vi "image queue to disk and to display queue_MD.vi"() -> ()   [LabVIEW 2012]
uses:
  <vilib>/Utility/VariantDataType/Type.ctl
  Custom Controls/file format type def.ctl
  GFG/GFGnumericGet.vi
  GFG/GFGbooleanGet.vi
  save images/save channels to raw bin files.vi
  save images/save channels to interleaved multi-tiff files.vi
  save images/save channels to separate multi-tiff files.vi
  save images/save channels to stacked multi-tiff files.vi
  save images/save channels to interleaved tiff series.vi
  save images/save channels to separate tiff series.vi
  save images/save channels to stacked tiff series.vi
  GFG/GFG library.lvlib
  <vilib>/Utility/VariantDataType/VariantType.lvlib
panel:
  out "error out 4":errorcluster
  out "error out 3":errorcluster
  out "error out 2":errorcluster
  out "# elements in image data queue":i32
  out "error out":errorcluster
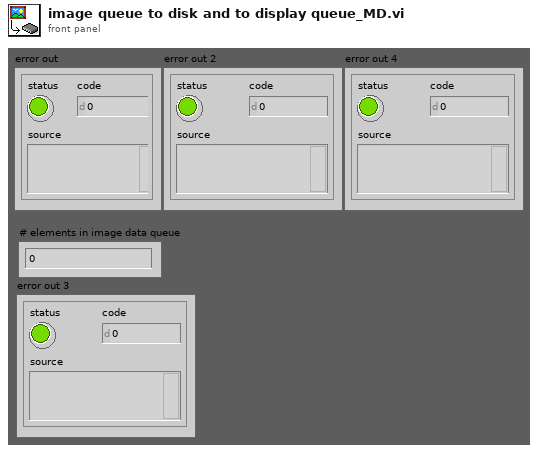
[diagram p1: front panel]
types:
  T1 = typedef "file format type def.ctl" = enum16{"16bit raw", "32bit raw", "16bit multi-tiff (interleave)", "16bit multi-tiff (separate)", "16bit multi-tiff (stacked)", "32bit multi-tiff (interleave)", "32bit multi-tiff (separate)", "32bit multi-tiff (stacked)", "16bit tiff series (interleave)", "16bit tiff series (separate)", "16bit tiff series (stacked)", "32bit tiff series (interleave)", "32bit tiff series (separate)", "32bit tiff series (stacked)"}
  T2 = cluster{"NewVal":bool, "Event Registration Refnum":refnum<event-registration>}
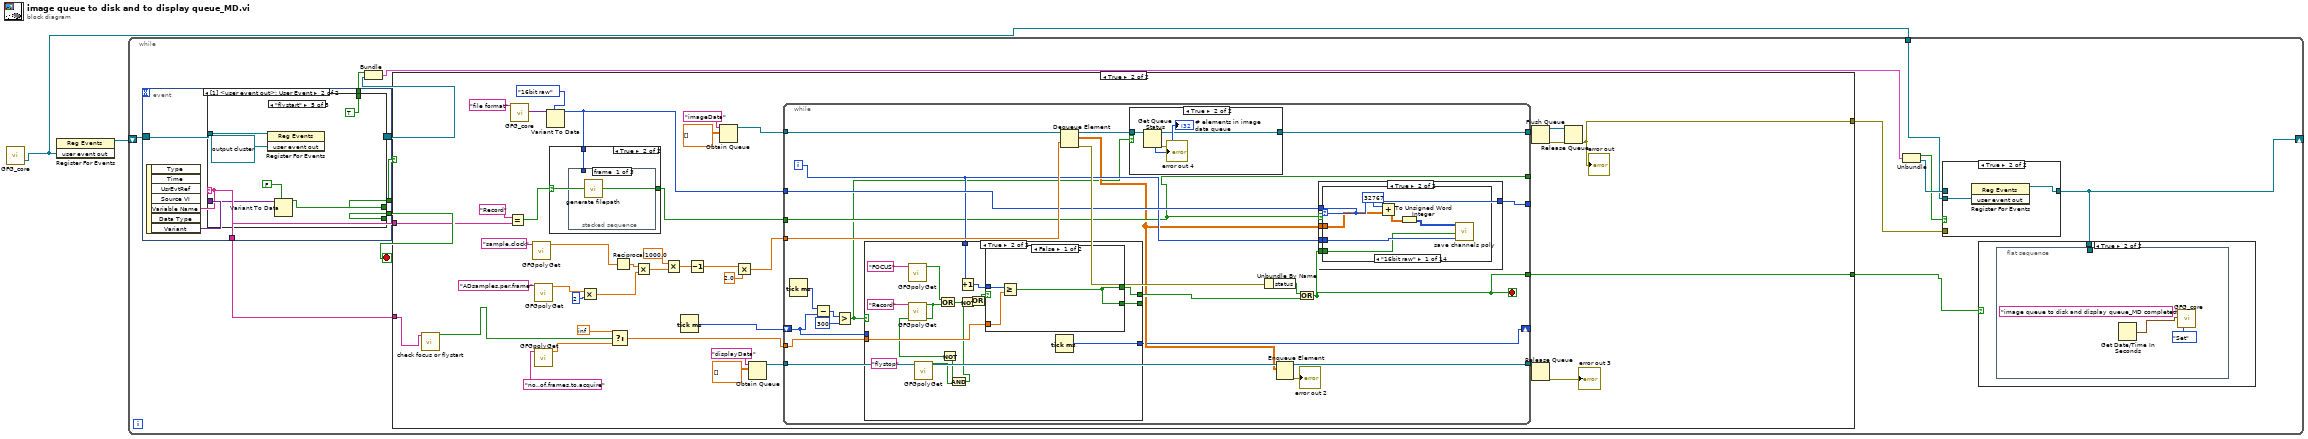
[diagram p0: block diagram]
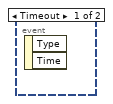
[diagram p4: hidden frame]
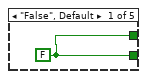
[diagram p5: hidden frame]
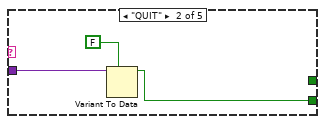
[diagram p6: hidden frame]
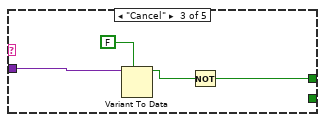
[diagram p7: hidden frame]
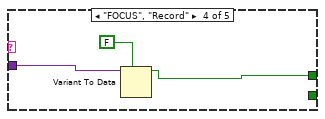
[diagram p8: hidden frame]
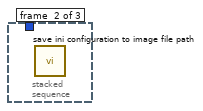
[diagram p11: hidden frame]
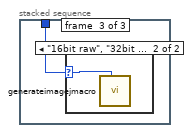
[diagram p12: hidden frame]
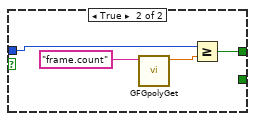
[diagram p16: hidden frame]
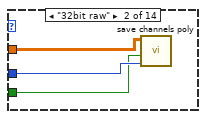
[diagram p18: hidden frame]
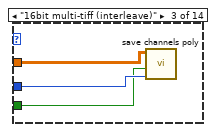
[diagram p19: hidden frame]
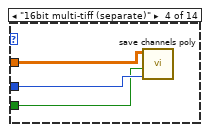
[diagram p20: hidden frame]
diagram:
  n1 = call "GFG_core.vi"() -> ("user event out"=w1:refnum<user-event>)  [unwired: 13 in, 6 out]
  n2 = register-events(w1) -> (reference out=w2:refnum<event-registration>)  [unwired: 2 in, 1 out]
  n3 = while {
    tunnel: w1 -> [w6]
    shift-right: [w4] -> _
    shift-left: w2 -> [w13]
    stop <- w15 stop-if-true
    n4 = event shown="[1] <user event out>: User Event" {
      selector: w13 -> [_ w24]
      dyn-events: [_ _] -> w11
      timeout: _ -> [_ _]
      tunnel: [_ w28] -> w14
      tunnel: [_ w27] -> w15
      tunnel: [_ w25] -> w5
      tunnel: [_ w23] -> w12
      event Timeout {
        n5 = event-data() -> ()  [unwired: 1 in, 2 out]
      }
      event User Event {
        n6 = event-data() -> ("Variable Name"=w25:string, "Variant"=w26:variant)  [unwired: 1 in, 5 out]
        n7 = case shown="\"flystart\"" w25 {
          tunnel: [w29 _ w33 w37 w43] -> w28
          tunnel: [w29 w30 _ _ _] -> w27
          tunnel: w26 -> [_ w32 w35 w38 w44]
          tunnel: w24 -> [_ _ _ _ w41]
          tunnel: [_ _ _ _ TRUE ("NewVal")] -> w23
          frame "False", Default {
            w29 = FALSE ("NewVal")
          }
          frame "QUIT" {
            n8 = Variant To Data(type=FALSE ("NewVal"), Variant=w32) -> (data=w30:bool)  [unwired: 1 in, 1 out]
          }
          frame "Cancel" {
            n9 = Variant To Data(type=FALSE ("NewVal"), Variant=w35) -> (data=w34:bool)  [unwired: 1 in, 1 out]
            n10 = Not(x=w34) -> (.not. x?=w33:bool)
          }
          frame "FOCUS", "Record" {
            n11 = Variant To Data(type=FALSE ("NewVal"), Variant=w38) -> (data=w37:bool)  [unwired: 1 in, 1 out]
          }
          frame "flystart" {
            n12 = register-events(reference=w41, refnum<user-event> refnum ("user event out")) -> ()  [unwired: 1 in, 2 out]
            n13 = Variant To Data(type=FALSE ("NewVal"), Variant=w44) -> (data=w43:bool)  [unwired: 1 in, 1 out]
          }
        }
      }
    }
    n14 = Bundle("NewVal"=w12, "Event Registration Refnum"=w11) -> (w9:T2)  [unwired: 1 in]
    n15 = case shown="True" w14 {
      tunnel: w5 -> [_ w64]
      tunnel: [_ w53] -> w10
      tunnel: w5 -> [_ w48]
      tunnel: [_ w46] -> w3
      frame False {
      }
      frame True {
        n16 = call "check focus or flystart.vi"("x"=w48) -> ("x .or. y?"=w47:bool)  [unwired: 10 in]
        n17 = Equal?(x="Record", y=w64) -> (x = y?=w58:bool)
        n18 = call "GFG_core.vi"("Variable Name in"="file format") -> ("Variant Out"=w60:variant)  [unwired: 12 in, 6 out]
        n19 = call-poly "GFGpolyGet.vi"("Variable Name in"="sample.clock" ("Tag in")) -> ("Numeric"=w71:dbl)  [unwired: 9 in, 1 out]
        n20 = call-poly "GFGpolyGet.vi"("Variable Name in"="ADsamples.per.frame" ("Tag in")) -> ("Numeric"=w77:dbl)  [unwired: 9 in, 1 out]
        n21 = call-poly "GFGpolyGet.vi"("Variable Name in"="no..of.frames.to.acquire" ("Tag in")) -> ("Numeric"=w50:dbl)  [unwired: 9 in, 1 out]
        n22 = Variant To Data(type=file_format_type_def."16bit raw" ("file format"), Variant=w60) -> (data=w56:T1)  [unwired: 1 in, 1 out]
        n23 = case shown="True" w58 {
          selector: w58 -> [w87 w89]
          tunnel: [w87 w89] -> w57
          tunnel: w56 -> [_ w88]
          frame False {
          }
          frame True {
            n24 = stacked-sequence {
              tunnel: w88 -> [_ _ w90]
              frame #0 {
                n25 = call "generate filepath.vi"() -> ()  [unwired: 12 in]
              }
              frame #1 {
                n26 = call "save ini configuration to image file path.vi"() -> ()  [unwired: 12 in]
              }
              frame #2 {
                n27 = case shown="\"16bit raw\", \"32bit raw\"" w90 {
                  selector: w90 -> [_ w91]
                  frame Default {
                  }
                  frame "16bit raw", "32bit raw" {
                    n28 = call "generateimagejmacro.vi"("file format"=w91) -> ()  [unwired: 11 in]
                  }
                }
              }
            }
          }
        }
        n29 = Multiply(x=w77, y=i8 2) -> (x*y=w70:dbl)
        n30 = Select(t=inf, s=w47, f=w50) -> (s? t:f=w49:dbl)
        n31 = Reciprocal(x=w71) -> (1/x=w76:dbl)
        n32 = Multiply(x=w76, y=w70) -> (x*y=w75:dbl)
        n33 = Multiply(x=1000.0, y=w75) -> (x*y=w73:dbl)
        n34 = Tick Count (ms)() -> (millisecond timer value=w55:u32)
        n35 = Decrement(x=w73) -> (x-1=w62:dbl)
        n36 = Obtain Queue(name (unnamed)="imageData", element data type=dbl[][] [] ("y backward image")) -> (queue out=w67:refnum<queue>)  [unwired: 3 in, 2 out]
        n37 = Multiply(x=w62, y=2.0 ("x-1")) -> (x*y=w66:dbl)
        n38 = Obtain Queue(name (unnamed)="displayData", element data type=dbl[][] [] ("y backward image")) -> (queue out=w84:refnum<queue>)  [unwired: 3 in, 2 out]
        n39 = while {
          tunnel: [w106] -> w82
          tunnel: w84 -> [w110]
          tunnel: [w114] -> w83
          tunnel: w49 -> [w112]
          tunnel: w66 -> [w108]
          tunnel: w67 -> [w109]
          tunnel: w57 -> [w102]
          tunnel: w56 -> [w105]
          tunnel: [w102] -> _
          tunnel: [w101] -> _
          shift-right: [w96] -> _
          shift-left: w55 -> [w95]
          tunnel: [w92] -> w46
          i -> [w103]
          stop <- w92 stop-if-true
          n40 = Tick Count (ms)() -> (millisecond timer value=w99:u32)
          n41 = Subtract(x=w99, y=w95) -> (x-y=w98:u32)
          n42 = Greater?(x=w98, y=u32 300) -> (0:w94:bool)
          n43 = case shown="True" w94 {
            tunnel: w112 -> [_ w137]
            tunnel: [_ w130] -> w104
            tunnel: w103 -> [_ w129]
            tunnel: [w120 w128] -> w96
            tunnel: w95 -> [w120 _]
            tunnel: [_ w127] -> _
            frame False {
            }
            frame True {
              n44 = call-poly "GFGpolyGet.vi"("Variable Name in"="FOCUS") -> ("Boolean"=w134:bool)  [unwired: 10 in]
              n45 = call-poly "GFGpolyGet.vi"("Variable Name in"="Record") -> ("Boolean"=w123:bool)  [unwired: 10 in]
              n46 = call-poly "GFGpolyGet.vi"("Variable Name in"="flystop") -> ("Boolean"=w124:bool)  [unwired: 10 in]
              n47 = Or(x=w134, y=w123) -> (x .or. y?=w133:bool)
              n48 = Not(x=w123) -> (.not. x?=w125:bool)
              n49 = And(x=w125, y=w124) -> (x .and. y?=w121:bool)
              n50 = Increment(x=w129) -> (x+1=w132:i32)
              n51 = Not(x=w133) -> (.not. x?=w131:bool)
              n52 = Or(x=w121, y=w131) -> (x .or. y?=w122:bool)
              n53 = case shown="False" w122 {
                tunnel: w137 -> [w140 _]
                tunnel: w132 -> [w139 w143]
                tunnel: [w138 w142] -> w130
                tunnel: [w138 _] -> w127
                frame False {
                  n54 = Greater Or Equal?(x=w139, y=w140) -> (x >= y?=w138:bool)
                }
                frame True {
                  n55 = call-poly "GFGpolyGet.vi"("Variable Name in"="frame.count") -> ("Numeric"=w141:dbl)  [unwired: 9 in, 1 out]
                  n56 = Greater Or Equal?(x=w143, y=w141) -> (x >= y?=w142:bool)
                }
              }
              n57 = Tick Count (ms)() -> (millisecond timer value=w128:u32)
            }
          }
          n58 = Dequeue Element(queue=w109, timeout in ms (-1)=w108) -> (queue out=w107:refnum<queue>, element=w100:dbl[][], error out=w111:errorcluster)  [unwired: 1 in, 1 out]
          n59 = case shown="True" w94 {
            tunnel: w107 -> [w115 w118]
            tunnel: [w115 w117] -> w106
            frame False {
            }
            frame True {
              n60 = Get Queue Status(queue=w118) -> (queue out=w117:refnum<queue>, error out=→"error out 4":errorcluster, # elements in queue=→"# elements in image data queue":i32)  [unwired: 2 in, 5 out]
            }
          }
          n61 = Unbundle By Name(w111) -> ("status"=w113:bool)
          n62 = Enqueue Element(queue=w110, element=w100) -> (queue out=w114:refnum<queue>, error out=→"error out 2":errorcluster)  [unwired: 2 in, 1 out]
          n63 = Or(x=w113, y=w104) -> (x .or. y?=w92:bool)
          n64 = case shown="True" w102 {
            tunnel: w103 -> [_ w148]
            tunnel: w92 -> [_ w147]
            tunnel: w105 -> [w145 w146]
            tunnel: w100 -> [_ w149]
            tunnel: [w145 w146] -> w101
            frame False {
            }
            frame True {
              n65 = case shown="\"16bit raw\"" w146 {
                tunnel: w149 -> [w151 w158 w161 w164 w167 w170 w173 w176 w179 w182 w185 w188 w191 w194]
                tunnel: w148 -> [w155 w157 w160 w163 w166 w169 w172 w175 w178 w181 w184 w187 w190 w193]
                tunnel: w147 -> [w154 w156 w159 w162 w165 w168 w171 w174 w177 w180 w183 w186 w189 w192]
                frame "16bit raw" {
                  n66 = Add(x=i16 32767, y=w151) -> (x+y=w153:dbl[][])
                  n67 = To Unsigned Word Integer(number=w153) -> (unsigned 16bit integer=w150:u16[][])
                  n68 = call-poly "save channels poly.vi"("frame number in"=w155, "last frame"=w154, "image data in (U16)"=w150) -> ()  [unwired: 9 in]
                }
                frame "32bit raw" {
                  n69 = call-poly "save channels poly.vi"("frame number in"=w157, "last frame"=w156, "image data in (U16)"=w158) -> ()  [unwired: 9 in]
                }
                frame "16bit multi-tiff (interleave)" {
                  n70 = call-poly "save channels poly.vi"("frame number in"=w160, "last frame"=w159, "image data in"=w161) -> ()  [unwired: 9 in]
                }
                frame "16bit multi-tiff (separate)" {
                  n71 = call-poly "save channels poly.vi"("frame number in"=w163, "last frame"=w162, "image data in"=w164) -> ()  [unwired: 9 in]
                }
                frame "16bit multi-tiff (stacked)" {
                  n72 = call-poly "save channels poly.vi"("frame number in"=w166, "last frame"=w165, "image data in"=w167) -> ()  [unwired: 9 in]
                }
                frame "32bit multi-tiff (interleave)" {
                  n73 = call-poly "save channels poly.vi"("frame number in"=w169, "last frame"=w168, "image data in"=w170) -> ()  [unwired: 9 in]
                }
                frame "32bit multi-tiff (separate)" {
                  n74 = call-poly "save channels poly.vi"("frame number in"=w172, "last frame"=w171, "image data in"=w173) -> ()  [unwired: 9 in]
                }
                frame "32bit multi-tiff (stacked)" {
                  n75 = call-poly "save channels poly.vi"("frame number in"=w175, "last frame"=w174, "image data in"=w176) -> ()  [unwired: 9 in]
                }
                frame "16bit tiff series (interleave)" {
                  n76 = call-poly "save channels poly.vi"("frame number in"=w178, "last frame"=w177, "image data in"=w179) -> ()  [unwired: 9 in]
                }
                frame "16bit tiff series (separate)" {
                  n77 = call-poly "save channels poly.vi"("frame number in"=w181, "last frame"=w180, "image data in"=w182) -> ()  [unwired: 9 in]
                }
                frame "16bit tiff series (stacked)" {
                  n78 = call-poly "save channels poly.vi"("frame number in"=w184, "last frame"=w183, "image data in"=w185) -> ()  [unwired: 9 in]
                }
                frame "32bit tiff series (interleave)" {
                  n79 = call-poly "save channels poly.vi"("frame number in"=w187, "last frame"=w186, "image data in"=w188) -> ()  [unwired: 9 in]
                }
                frame "32bit tiff series (separate)" {
                  n80 = call-poly "save channels poly.vi"("frame number in"=w190, "last frame"=w189, "image data in"=w191) -> ()  [unwired: 9 in]
                }
                frame "32bit tiff series (stacked)" {
                  n81 = call-poly "save channels poly.vi"("frame number in"=w193, "last frame"=w192, "image data in"=w194) -> ()  [unwired: 9 in]
                }
              }
            }
          }
        }
        n82 = Release Queue(queue=w83) -> (error out=→"error out 3":errorcluster)  [unwired: 2 in, 2 out]
        n83 = Flush Queue(queue=w82) -> (queue out=w81:refnum<queue>, error out=w80:errorcluster)  [unwired: 1 in, 1 out]
        n84 = Release Queue(queue=w81, error in (no error)=w80) -> (error out=w53:errorcluster)  [unwired: 1 in, 2 out]
        "error out" <- w53
      }
    }
    n85 = Unbundle(w9) -> ("NewVal"=w7:bool, "Event Registration Refnum"=w8:refnum<event-registration>)
    n86 = case shown="True" w7 {
      tunnel: [w20 w22] -> w4
      tunnel: w6 -> [_ w21]
      tunnel: w10 -> [_ _]
      tunnel: w8 -> [w20 _]
      frame False {
      }
      frame True {
        n87 = register-events(w21) -> (reference out=w22:refnum<event-registration>)  [unwired: 2 in, 1 out]
      }
    }
    n88 = case shown="True" w3 {
      tunnel: w4 -> [_ w16]
      frame False {
      }
      frame True {
        n89 = flat-sequence {
          tunnel: w16 -> [_]
          frame #0 {
            n90 = Get Date/Time In Seconds() -> (seconds since 1Jan1904=w17:timestamp)
            n91 = call "GFG_core.vi"("Variable Name in"="image queue to disk and display queue_MD completed", "Variant in"=w17, "Action"=enum16{"Init", "Set", "Get"}."Set") -> ()  [unwired: 10 in, 7 out]
          }
        }
      }
    }
  }
